vi "101_HowToConnect.vi"() -> ()   [LabVIEW 2009]
uses:
  <instrlib>/Zurich Instruments LabOne/Zurich Instruments LabOne.lvlib
panel:
  out "Connected?":bool
  out "Message":string
  out "Error Out":errorcluster
  in  "Address":string="DEV"
  # "How to connect to an Instrument\nThis VI shows how to connect to an instrument.\n\nSee block diagram for the  VI description.\n\nRequirements: Any Zurich Instrument Product\n\nTo run\n1- Type the Device ID in the form of DEVXXXX as indicated on the back panel of the instrument itself.\n2- Run the VI\n* If the connection is successful, the \"connected?\" boolean lights up green. \n\nTested Devices:\n- HF2LI\n- UHFLI\n- MFLI\n\n(c) Zurich Instruments.  ALL RIGHTS RESERVED."
  # "Note on the Message: \nThe API version and revision should match with the Data Server for the best performance. \n\nSee:\nhttps://docs.zhinst.com/labone_programming_manual/labview.html#pm.labview.installation"
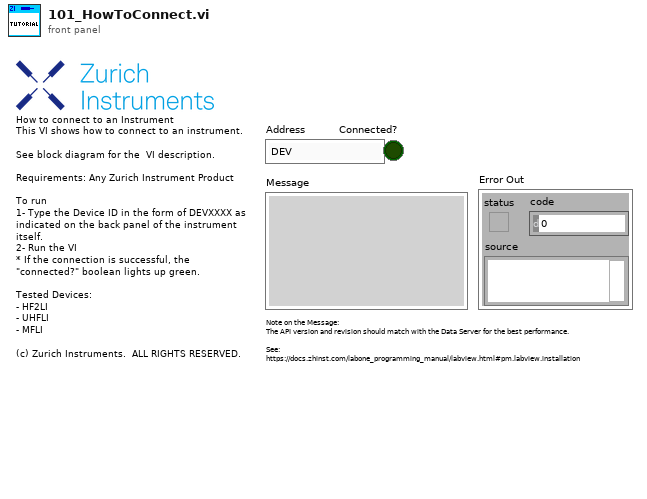
[diagram p1: front panel]
types:
  T1 = typedef "Zurich Instruments LabOne.lvlib/ziTypeHandle.ctl" = cluster{"handleValid":bool, "Conn":u64, "Path Prefix":string, "Handle":u64, "Connected":bool, "Clockbase(s)":dbl}
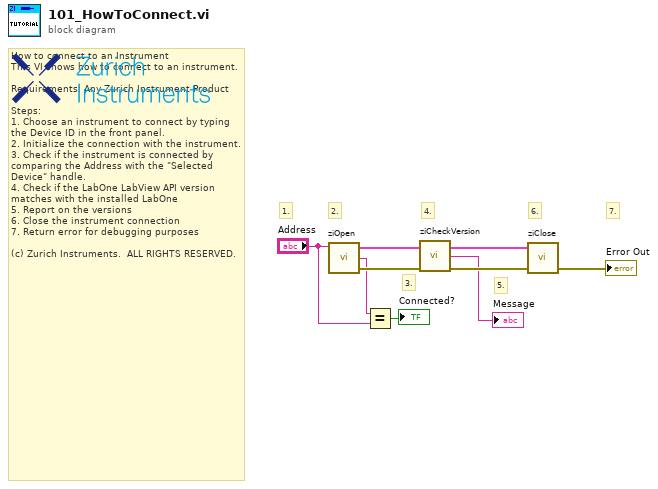
[diagram p0: block diagram]
diagram:
  # "5."
  # "3."
  # "2."
  # "1."
  # "7."
  # "6."
  # "4."
  # "How to connect to an Instrument\nThis VI shows how to connect to an instrument.\n\nRequirements: Any Zurich Instrument Product\n\nSteps:\n1. Choose an instrument to connect by typing the Device ID in the front panel.\n2. Initialize the connection with the instrument.\n3. Check if the instrument is connected by comparing the Address with the \"Selected Device\" handle. \n4. Check if the LabOne LabView API version matches with the installed LabOne  \n5. Report on the versions\n6. Close the instrument connection\n7. Return error for debugging purposes \n\n(c) Zurich Instruments.  ALL RIGHTS RESERVED."
  n1 = call <instrlib>:"ziOpen.vi"("Address"="Address") -> ("Error Out"=w8:errorcluster, "Selected Device"=w2:string, "HandleOut"=w9:T1)  [unwired: 1 in, 2 out]
  n2 = Equal?(x=w2, y="Address") -> (x = y?=→"Connected?":bool)
  n3 = call <instrlib>:"ziCheckVersion.vi"("Handle In"=w9, "Error In"=w8) -> ("Handle Out"=w7:T1, "Message"=→"Message":string, "Error Out"=w6:errorcluster)  [unwired: 11 in]
  n4 = call <instrlib>:"ziClose.vi"("Error In"=w6, "Handle In"=w7) -> ("Error Out"=→"Error Out":errorcluster)  [unwired: 2 in, 1 out]
